vi "Get Folder.vi"(8 "error in":errorcluster) -> (0 "error out":errorcluster, 3 "dup path":path)   [LabVIEW 2015, in "Logger.lvlib"]
uses:
  Logger.lvlib
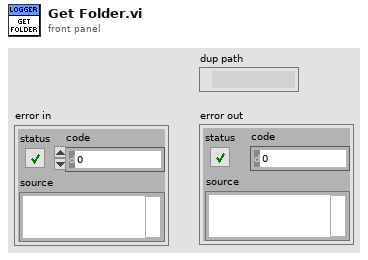
[diagram p1: front panel]
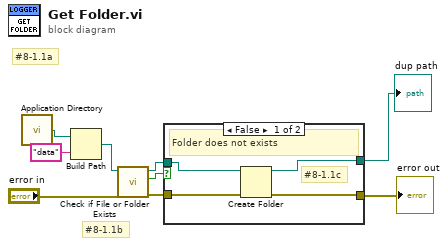
[diagram p0: block diagram]
diagram:
  # "#8-1.1b"
  # "#8-1.1a"
  n1 = call <vilib>:"Application Directory.vi"() -> ("Application Directory"=w8:path)
  n2 = Build Path(base path=w8, name or relative path="data") -> (appended path=w6:path)
  n3 = call <vilib>:"Check if File or Folder Exists.vi"("error in (no error)"="error in", "path"=w6) -> ("error out"=w4:errorcluster, "file or folder exists?"=w9:bool, "dup path"=w2:path)  [unwired: 7 in]
  n4 = case shown="False" w9 {
    tunnel: w4 -> [w12 w15]
    tunnel: [w11 w15] -> w3
    tunnel: w2 -> [w13 w14]
    tunnel: [w10 w14] -> w1
    frame False {
      # "#8-1.1c"
      # "Folder does not exists"
      n5 = Create Folder(path (use dialog)=w13, error in=w12) -> (created path=w10:path, error out=w11:errorcluster)  [unwired: 1 in, 1 out]
    }
    frame True {
      # "Folder exists"
    }
  }
  "error out" <- w3
  "dup path" <- w1
